vi "SetUSB5DoSampleMode.vi"(8 "错误输入（无错误）":errorcluster, 10 "DoSampleMode":u8(ring)=1 items=["PcBufferedInfinite", "NCycle"], 11 "DevIndex":i32) -> (0 "错误输出":errorcluster, 3 "DevIndex Out":i32)   [LabVIEW 2020]
uses:
  lib/x64/USB5000.dll
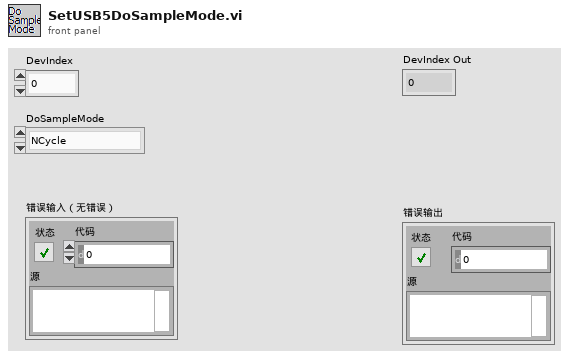
[diagram p1: front panel]
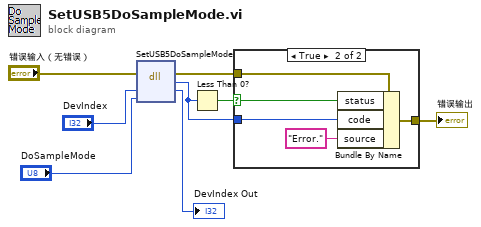
[diagram p0: block diagram]
diagram:
  n1 = dll-call lib="C:/Users/phosense/Downloads/USB-5000/USB-5000_LabVIEW/lib/x64/USB5000.dll" fn="SetUSB5DoSampleMode"(error in="错误输入（无错误）", "DevIndex"="DevIndex", "DoSampleMode"="DoSampleMode") -> (error out=w4:errorcluster, "返回类型"=w3:i32, "DevIndex"=→"DevIndex Out":i32)  [unwired: 3 in, 1 out]
  n2 = Less Than 0?(x=w3) -> (x < 0?=w5:bool)
  n3 = case shown="True" w5 {
    selector: w5 -> [_ w10]
    tunnel: [w9 w12] -> w2
    tunnel: w3 -> [_ w14]
    tunnel: w4 -> [w9 w11]
    frame False {
    }
    frame True {
      n4 = Bundle By Name(cluster=w11, "status"=w10, "code"=w14, "source"="Error." ("error message (\"\")")) -> (w12:errorcluster)
    }
  }
  "错误输出" <- w2
